vi "Write Forecast Data Long DVR.vi"(8 "error in":errorcluster, 10 "ForecastData":T1, 11 "EMS Generic in":refnum<class "EMS Generic.lvclass">) -> (0 "error out":errorcluster, 3 "EMS Generic out":refnum<class "EMS Generic.lvclass">)   [LabVIEW 2018, in "EMS Generic Actor.lvlib" / "EMS Generic.lvclass"]
uses:
  EMS Generic.lvclass
  <vilib>/ORNL/CSEISMIC DDS/CSEISMIC DDS Base/Data Types/ForecastData_Data.ctl
  <vilib>/ORNL/CSEISMIC DDS/CSEISMIC DDS Base/Data Types/Controls/DeviceID.ctl
  EMS Generic.lvclass/EMS Generic.ctl
  <vilib>/ORNL/CSEISMIC DDS/CSEISMIC DDS Base/CSEISMIC DDS.lvclass
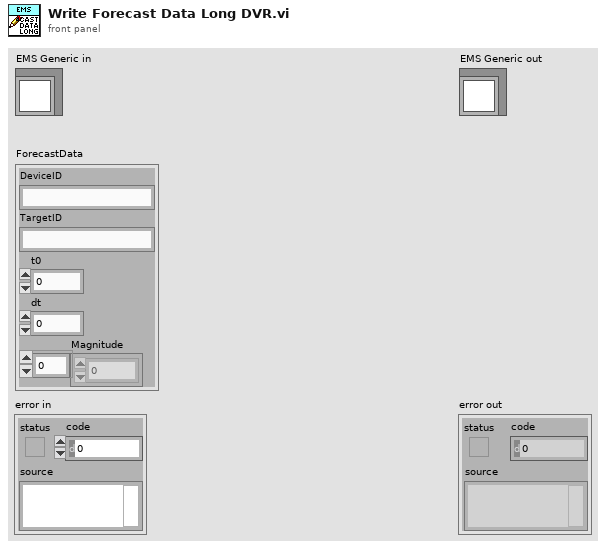
[diagram p1: front panel]
types:
  T1 = typedef "CSEISMIC DDS.lvlib/CSEISMIC DDS.lvclass/ForecastData_Data.ctl" = cluster{"DeviceID":T2, "TargetID":T2, "t0":dbl, "dt":dbl, "Magnitude":dbl[]}
  T2 = typedef "CSEISMIC DDS.lvlib/CSEISMIC DDS.lvclass/DeviceID.ctl" = string
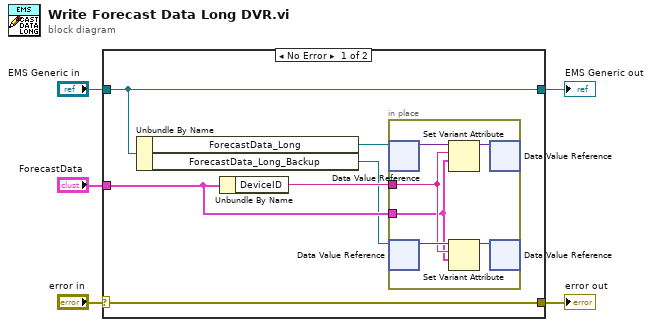
[diagram p0: block diagram]
diagram:
  n1 = case shown="No Error" "error in" {
    selector: "error in" -> [w11 w19]
    tunnel: [w11 w19] -> w4
    tunnel: [w10 w18] -> w2
    tunnel: "EMS Generic in" -> [w10 w18]
    tunnel: "ForecastData" -> [w8 _]
    frame No Error {
      n2 = Unbundle By Name(w10) -> ("ForecastData_Long"=w7:refnum<data-value>, "ForecastData_Long_Backup"=w6:refnum<data-value>)
      n3 = Unbundle By Name(w8) -> ("DeviceID"=w9:T2)
      n4 = in-place {
        in-place-border: w9 -> [w13]
        in-place-border: w8 -> [w12]
        n5 = in-place-dvr #1(w7) -> (w17:variant)  [unwired: 1 out]
        n6 = in-place-dvr #2(w6) -> (w15:variant)  [unwired: 1 out]
        n7 = Set Variant Attribute(Variant=w17, name=w13, value=w12) -> (Variant out=w16:variant)  [unwired: 1 in, 2 out]
        n8 = Set Variant Attribute(Variant=w15, name=w13, value=w12) -> (Variant out=w14:variant)  [unwired: 1 in, 2 out]
        n9 = in-place-dvr #1(w16) -> ()  [unwired: 2 out]
        n10 = in-place-dvr #2(w14) -> ()  [unwired: 2 out]
      }
    }
    frame Error {
    }
  }
  "error out" <- w4
  "EMS Generic out" <- w2
